vi "GMLAN ReadFailureRecordData.vi"   [LabVIEW 2019, in "GMLAN.lvlib"]
uses:
  GMLAN.lvlib
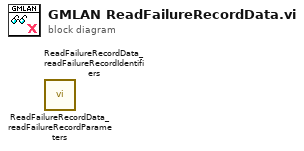
[diagram p0: block diagram]
diagram:
  n1 = call "ReadFailureRecordData_readFailureRecordParameters.vi"() -> ()  [unwired: 8 in, 4 out]
  n2 = call "ReadFailureRecordData_readFailureRecordIdentifiers.vi"() -> ()  [unwired: 8 in, 4 out]
